vi "Reset Node.vi"(8 "Error In":errorcluster, 10 "Node-ID":u8, 11 "ICommunicate":refnum<class "ICommunicate.lvclass">) -> (0 "Error Out":errorcluster)   [LabVIEW 2024, in "Network Mangement.lvclass"]
uses:
  Network Mangement.lvclass
  HAL/Source/Interfaces/ICommunicate/ICommunicate.lvclass
  source/CANopen Message/CANopen Message.lvclass
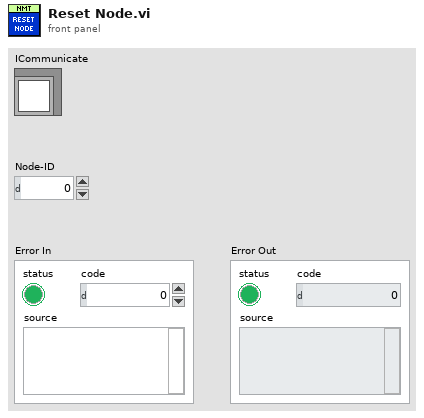
[diagram p1: front panel]
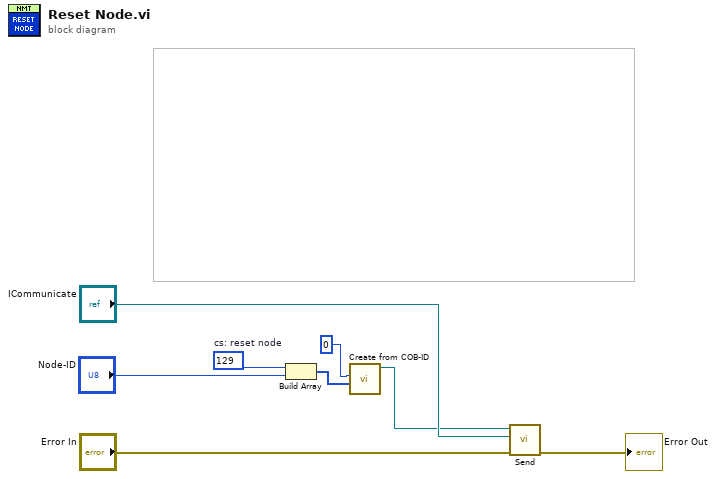
[diagram p0: block diagram]
diagram:
  w6 = u8 129  # cs: reset node
  n1 = Build Array(w6, "Node-ID") -> (w4:u8[])
  n2 = call "Create from COB-ID.vi"("Data"=w4, "COB-ID"=u32 0) -> ("CANopen Message out"=w7:refnum<class "CANopen Message.lvclass">)  [unwired: 9 in]
  n3 = call "Send.vi"("error in"="Error In", "ICommunicate"="ICommunicate", "CANopen Message in"=w7) -> ("error out"=→"Error Out":errorcluster)  [unwired: 7 in, 1 out]
